vi "Objects to table.vi"(8 "error in (no error)":errorcluster, 10 "Table Index":i32, 11 "object ref in":T1) -> (0 "error out":errorcluster, 2 "table":string[][](array[string]), 3 "object ref out":T1)   [LabVIEW 2014, in "Table Manager.lvlib" / "Table Manager.lvclass"]
doc: "Gets the table from the Objects Cluster"
uses:
  Table Manager.lvclass
  object ref.ctl
  Configuration Editor/Classes/Engine Parent/Engine Parent Editor Node.lvclass
  Configuration Editor/Classes/Module editor node/module editor node.lvclass
  Configuration Editor/Classes/Engine Parent/read engine configuration.vi
  <vilib>/NI/Module Execution Interface/Engine Configuration/engine configuration.lvclass
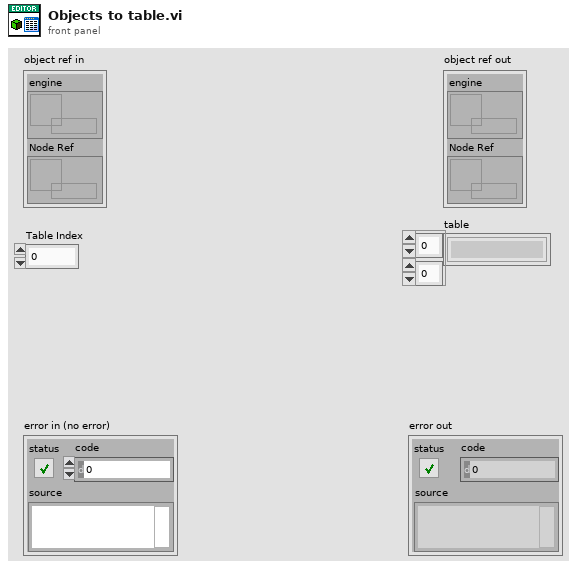
[diagram p1: front panel]
types:
  T1 = typedef "Table Manager.lvlib/Table Manager.lvclass/object ref.ctl" = cluster{"engine":refnum<data-value>, "Node Ref":refnum<data-value>}
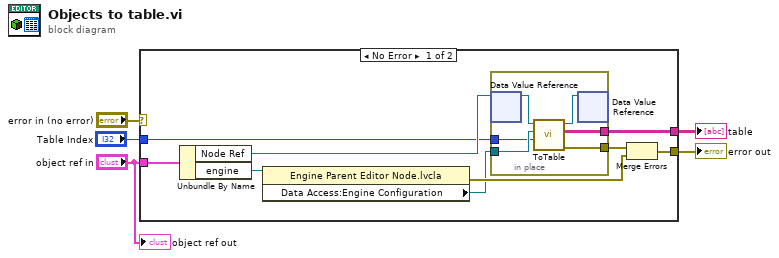
[diagram p0: block diagram]
diagram:
  n1 = case shown="No Error" "error in (no error)" {
    selector: "error in (no error)" -> [_ w21]
    tunnel: [w9 _] -> w5
    tunnel: "object ref in" -> [w13 _]
    tunnel: [w11 w21] -> w2
    tunnel: "Table Index" -> [w6 _]
    frame No Error {
      n2 = Unbundle By Name(w13) -> ("Node Ref"=w8:refnum<data-value>, "engine"=w14:refnum<data-value>)
      n3 = property class="Engine Parent Editor Node.lvcla"(reference=w14) -> (error out=w12:errorcluster, "Data Access:Engine Configuration"=w10:refnum<class "engine configuration.lvclass">)  [unwired: 1 in, 1 out]
      n4 = in-place {
        in-place-border: w10 -> [w20]
        in-place-border: [w19] -> w9
        in-place-border: [w16] -> w7
        in-place-border: w6 -> [w15]
        n5 = in-place-dvr #1(w8) -> (w18:refnum<class "module editor node.lvclass">)  [unwired: 1 out]
        n6 = call-dynamic "ToTable.vi"("Table Index"=w15, "variant"=w20, "node in"=w18) -> ("error out"=w16:errorcluster, "table"=w19:string[][], "node in out"=w17:refnum<class "module editor node.lvclass">)  [unwired: 5 in, 1 out]
        n7 = in-place-dvr #1(w17) -> ()  [unwired: 2 out]
      }
      n8 = Merge Errors(w7, w12) -> (w11:errorcluster)
    }
    frame Error {
    }
  }
  "table" <- w5
  "error out" <- w2
  "object ref out" <- "object ref in"
